vi "ChooChooLoop.vi"(8 "error in":errorcluster) -> ()   [LabVIEW 2013]
uses:
  Choo Choo State.ctl
  <vilib>/Rock Robotics/WPI/DigitalInput/WPI_DigitalInputDevRef.ctl
  <vilib>/Rock Robotics/SystemInterfaces/DIO/FPGA_DIOChannel.ctl
  <vilib>/Rock Robotics/SystemInterfaces/Typedef/FPGA_TypedefDigitalModule.ctl
  <vilib>/Rock Robotics/WPI/Encoder/WPI_EncoderDevRef.ctl
  <vilib>/Rock Robotics/SystemInterfaces/Encoder/FPGA_EncoderIdx.ctl
  <vilib>/Rock Robotics/SystemInterfaces/Counter/FPGA_CounterCtrSystemIndex.ctl
  <vilib>/Rock Robotics/WPI/Encoder/WPI_EncoderType.ctl
  <vilib>/Rock Robotics/WPI/MotorControl/WPI_MotorControlDeviceRef.ctl
  <vilib>/Rock Robotics/SystemInterfaces/DIO/FPGA_DIOPWMChannel.ctl
  <vilib>/Rock Robotics/WPI/PWM/WPI_PWMDeadband.ctl
  <vilib>/Rock Robotics/WPI/CAN/Jaguar/SubVIs/WPI_CANJaguar_ControlMode.ctl
  <vilib>/Rock Robotics/WPI/PWM/WPI_PWMTransform_ConPane.ctl
  <vilib>/Rock Robotics/WPI/Joystick/WPI_JoystickDeviceEnum.ctl
  <vilib>/Rock Robotics/WPI/SafetyOutput/WPI_SafetyOutputConfigMenu.ctl
  Robot Global Data.vi
  <vilib>/Rock Robotics/WPI/MotorControl/WPI_MotorControlSafetyCheck.vi
  <vilib>/Rock Robotics/Network Tables/SD Write String.vi
panel:
  in  "Timeout (ms)":i32=3000
  in  "Choo Choo Output":dbl=1.0
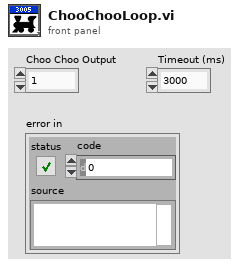
[diagram p1: front panel]
types:
  T1 = typedef "WPI_JoystickDeviceEnum.ctl" = enum16{"USB 1", "USB 2", "USB 3", "USB 4", "Kinect 1", "Kinect 2"}
  T2 = typedef "WPI_DigitalInputDevRef.ctl" = cluster{"DevStatus":errorcluster, "DIO Channel":T3, "Digital Module":T4}
  T3 = typedef "FPGA_DIOChannel.ctl" = enum8{"DIO 1", "DIO 2", "DIO 3", "DIO 4", "DIO 5", "DIO 6", "DIO 7", "DIO 8", "DIO 9", "DIO 10", "DIO 11", "DIO 12", "DIO 13", "DIO 14", "Invalid"}
  T4 = typedef "FPGA_TypedefDigitalModule.ctl" = enum16{"Digital Module 1", "Digital Module 2"}
  T5 = typedef "WPI_EncoderDevRef.ctl" = cluster{"DevStatus":errorcluster, "EncoderIndex":T6, "CounterIndex":T7, "DistancePerCount":dbl, "Decoding Type":T8}
  T6 = typedef "FPGA_EncoderIdx.ctl" = enum8{"Enc 0", "Enc 1", "Enc 2", "Enc 3", "Invalid"}
  T7 = typedef "FPGA_CounterCtrSystemIndex.ctl" = enum8{"Ctr 0", "Ctr 1", "Ctr 2", "Ctr 3", "Ctr 4", "Ctr 5", "Ctr 6", "Ctr 7", "Invalid"}
  T8 = typedef "WPI_EncoderType.ctl" = enum16{"1x", "2x", "4x"}
  T9 = typedef "WPI_MotorControlDeviceRef.ctl" = cluster{"DeviceStatus":errorcluster, "Type":enum16{"PWM", "CAN"}, "PWM":cluster{"Digital Module":T4, "PWM Channel":T10, "DeadBand":T11}, "CAN":cluster{"Device Number":u8, "Control Mode":T12, "Semaphore":T13, "Max Vout":dbl}, "Invert":bool, "TransformRef":T14, "InvTransformRef":T14}
  T10 = typedef "FPGA_DIOPWMChannel.ctl" = enum8{"PWM 1", "PWM 2", "PWM 3", "PWM 4", "PWM 5", "PWM 6", "PWM 7", "PWM 8", "PWM 9", "PWM 10", "Invalid"}
  T11 = typedef "WPI_PWMDeadband.ctl" = cluster{"Name":string, "maxPositivePwm":i32, "minPositivePwm":i32, "centerPwm":i32, "maxNegativePwm":i32, "minNegativePwm":i32, "angularRange":u16}
  T12 = typedef "WPI_CANJaguar_ControlMode.ctl" = enum8{"Percent VBus", "Current", "Speed", "Position", "Voltage"}
  T13 = typedef "Semaphore RefNum" = refnum<k1>
  T14 = typedef "WPI_PWMTransform_ConPane.ctl" = refnum<vi>
  T15 = cluster{"Ball Detect":T2, "CC Switch":T2, "Encoder":T5, "CCMotor":T9}
  T16 = typedef "Choo Choo State.ctl" = enum16{"Idle", "Check For Ball", "Drive Motor", "Delay", "Check Status", "Stop Motor"}
  T17 = typedef "WPI_JoystickDevRef.ctl" = cluster{"Device":T1}
  T18 = typedef "WPI_SafetyOutputConfigMenu.ctl" = enum16{"Enable", "Disable"}
  T19 = typedef "WPI_JoystickButtonState.ctl" = cluster{"Button 1":bool, "Button 2":bool, "Button 3":bool, "Button 4":bool, "Button 5":bool, "Button 6":bool, "Button 7":bool, "Button 8":bool, "Button 9":bool, "Button 10":bool, "Button 11":bool, "Button 12":bool}
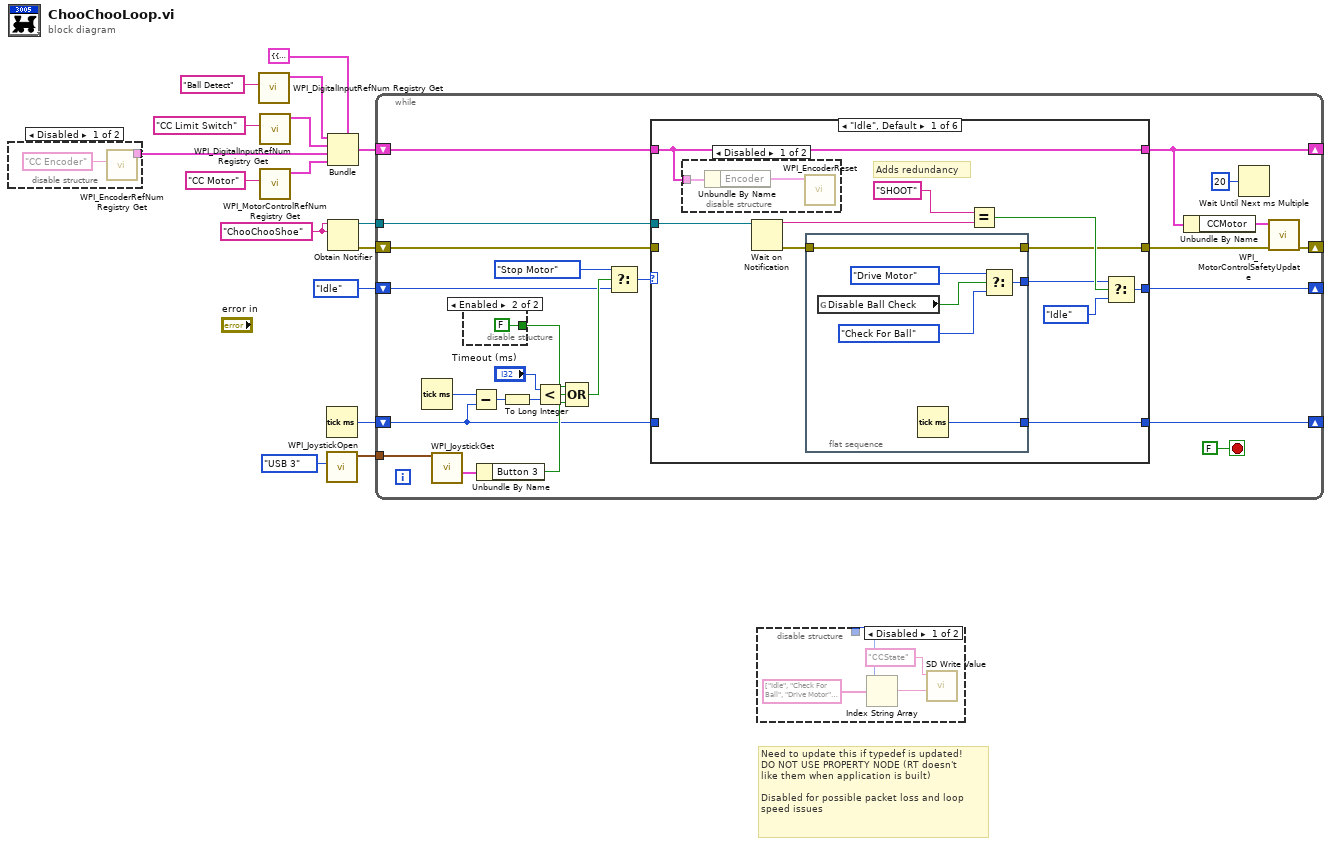
[diagram p0: block diagram]
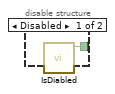
[diagram p4: hidden frame]
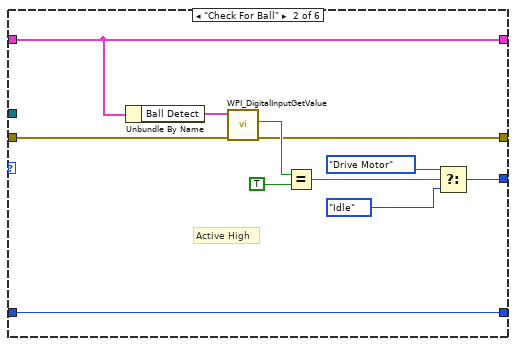
[diagram p6: hidden frame]
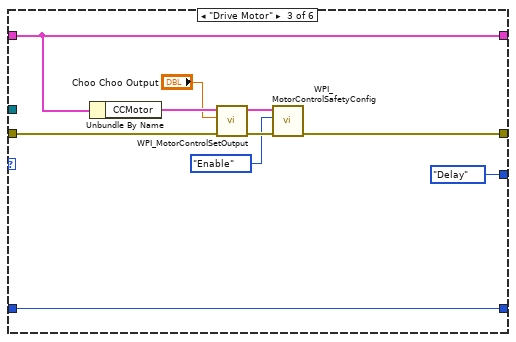
[diagram p7: hidden frame]
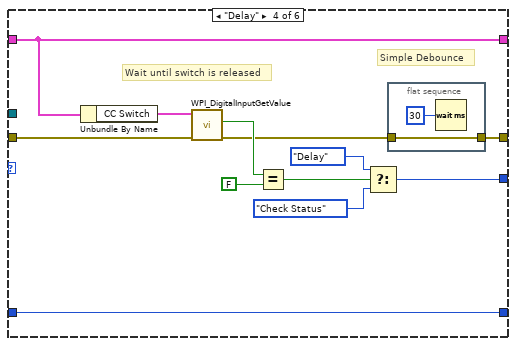
[diagram p8: hidden frame]
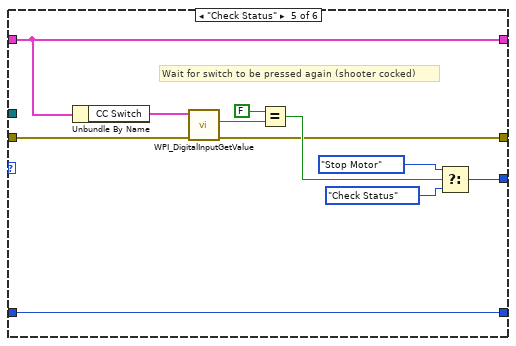
[diagram p9: hidden frame]
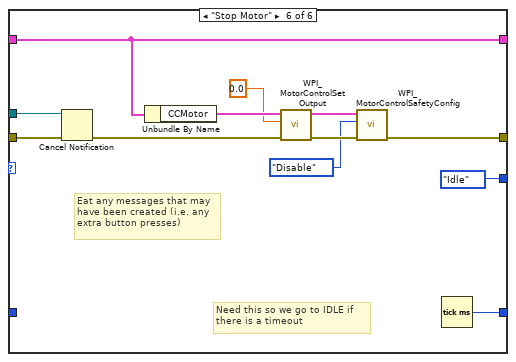
[diagram p10: hidden frame]
diagram:
  w10 = "ChooChooShoe" ("name (unnamed)")
  # "Need to update this if typedef is updated! \nDO NOT USE PROPERTY NODE (RT doesn't\nlike them when application is built)\n\nDisabled for possible packet loss and loop\nspeed issues"
  n1 = disable-structure shown="Disabled" {
    disable-tunnel: [w18 _] -> w11
    frame Disabled {
      n2 = call <vilib>:"WPI_EncoderRefNum Registry Get.vi"("refnum name"="CC Encoder") -> ("EncoderDevRef"=w18:T5)  [unwired: 9 in, 1 out]
    }
    frame Enabled {
    }
  }
  n3 = call <vilib>:"WPI_DigitalInputRefNum Registry Get.vi"("refnum name"="Ball Detect") -> ("DigitalInputDevRef"=w16:T2)  [unwired: 9 in, 1 out]
  n4 = call <vilib>:"WPI_DigitalInputRefNum Registry Get.vi"("refnum name"="CC Limit Switch") -> ("DigitalInputDevRef"=w13:T2)  [unwired: 9 in, 1 out]
  n5 = call <vilib>:"WPI_MotorControlRefNum Registry Get.vi"("refnum name"="CC Motor") -> ("MotorControlDevRef"=w9:T9)  [unwired: 9 in, 1 out]
  n6 = Tick Count (ms)() -> (millisecond timer value=w3:u32)
  n7 = call <vilib>:"WPI_JoystickOpen.vi"("JoystickDevice"=WPI_JoystickDeviceEnum."USB 3") -> ("JoystickDevRef"=w2:T17)  [unwired: 10 in]
  n8 = Bundle(cluster=T15 {"Ball Detect"={"DevStatus"={"status"=FALSE, "code"=0, "source"=""}, "DIO Channel"=enum."DIO 1", "Digital Module"=enum."Digital Module 1"}, "CC Switch"={"DevStatus"={"status"=FALSE, "code"=0, "source"=""}, "DIO Channel"=enum."DIO 1", "Digital Module"=enum."Digital Module 1"}, "Encoder"={"DevStatus"={"status"=FALSE, "code"=0, "source"=""}, "EncoderIndex"=enum."Enc 0", "CounterIndex"=enum."Ctr 0", "DistancePerCount"=0.0, "Decoding Type"=enum."1x"}, "CCMotor"={"DeviceStatus"={"status"=FALSE, "code"=0, "source"=""}, "Type"=enum."PWM", "PWM"={"Digital Module"=enum."Digital Module 1", "PWM Channel"=enum."PWM 1", "DeadBand"={"Name"="", "maxPositivePwm"=0, "minPositivePwm"=0, "centerPwm"=0, "maxNegativePwm"=0, "minNegativePwm"=0, "angularRange"=0}}, "CAN"={"Device Number"=0, "Control Mode"=enum."Percent VBus", "Semaphore"=refnum, "Max Vout"=0.0}, "Invert"=FALSE, "TransformRef"=refnum, "InvTransformRef"=refnum}}, "Ball Detect"=w16, "CC Switch"=w13, "Encoder"=w11, "CCMotor"=w9) -> (w7:T15)
  n9 = Obtain Notifier(name (unnamed)=w10, notification data type=w10) -> (notifier out=w6:refnum<notifier>, error out=w5:errorcluster)  [unwired: 2 in, 1 out]
  n10 = while {
    shift-right: [w36] -> _
    shift-left: w7 -> [w41]
    shift-right: [w33] -> _
    shift-left: Choo_Choo_State."Idle" -> [w24]
    tunnel: w6 -> [w40]
    shift-right: [w37] -> _
    shift-left: w5 -> [w39]
    shift-right: [w34] -> _
    shift-left: w3 -> [w20]
    tunnel: w2 -> [w21]
    stop <- FALSE stop-if-true
    n11 = Tick Count (ms)() -> (millisecond timer value=w31:u32)
    n12 = call <vilib>:"WPI_JoystickGet.vi"("JoystickDevRef"=w21) -> ("Buttons"=w19:T19)  [unwired: 4 in, 2 out]
    n13 = disable-structure shown="Enabled" {
      disable-tunnel: [w44 FALSE ("Is Disabled?")] -> w27
      frame Disabled {
        n14 = call "IsDiabled.vi"() -> ("Is Disabled?"=w44:bool)  [unwired: 11 in]
      }
      frame Enabled {
      }
    }
    n15 = Subtract(x=w31, y=w20) -> (x-y=w30:u32)
    n16 = Unbundle By Name(w19) -> ("Button 3"=w22:bool)
    n17 = To Long Integer(number=w30) -> (32bit integer=w25:i32)
    n18 = Less?(x="Timeout (ms)", y=w25) -> (x < y?=w28:bool)
    n19 = Compound Arithmetic op=OR(w27, w28, w22) -> (w26:bool)
    n20 = Select(t=Choo_Choo_State."Stop Motor", s=w26, f=w24) -> (s? t:f=w23:T16)
    n21 = case shown="\"Idle\", Default" w23 {
      tunnel: w41 -> [w51 w75 w85 w97 w110 w122]
      tunnel: [w51 w75 w85 w97 w110 w122] -> w36
      tunnel: w40 -> [w56 _ _ _ _ w111]
      tunnel: [w52 w70 Choo_Choo_State."Delay" w92 w103 Choo_Choo_State."Idle"] -> w33
      tunnel: [w47 w66 w78 w87 w101 w116] -> w38
      tunnel: w39 -> [_ w73 w82 w95 w102 w120]
      tunnel: w20 -> [_ w65 w76 w86 w100 _]
      tunnel: [w46 w65 w76 w86 w100 w113] -> w34
      frame "Idle", Default {
        # "Adds redundancy"
        n22 = disable-structure shown="Disabled" {
          disable-tunnel: w51 -> [w64 _]
          frame Disabled {
            n23 = Unbundle By Name(w64) -> ("Encoder"=w63:T5)
            n24 = call <vilib>:"WPI_EncoderReset.vi"("EncoderDevRef"=w63) -> ()  [unwired: 9 in, 2 out]
          }
          frame Enabled {
          }
        }
        n25 = Wait on Notification(notifier=w56) -> (notification=w54:string, error out=w48:errorcluster)  [unwired: 3 in, 2 out]
        n26 = flat-sequence {
          tunnel: [w62] -> w49
          tunnel: w48 -> [w58]
          tunnel: [w58] -> w47
          tunnel: [w57] -> w46
          frame #0 {
            n27 = global read "Robot Global Data.vi" "Disable Ball Check"() -> (w59:bool)
            n28 = Tick Count (ms)() -> (millisecond timer value=w57:u32)
            n29 = Select(t=Choo_Choo_State."Drive Motor", s=w59, f=Choo_Choo_State."Check For Ball") -> (s? t:f=w62:T16)
          }
        }
        n30 = Equal?(x="SHOOT" ("name (unnamed)"), y=w54) -> (x = y?=w53:bool)
        n31 = Select(t=w49, s=w53, f=Choo_Choo_State."Idle") -> (s? t:f=w52:T16)
      }
      frame "Check For Ball" {
        # "Active High"
        n32 = Unbundle By Name(w75) -> ("Ball Detect"=w74:T2)
        n33 = call <vilib>:"WPI_DigitalInputGetValue.vi"("error in (no error)"=w73, "DigitalInputDevRef"=w74) -> ("error out"=w66:errorcluster, "Value"=w72:bool)  [unwired: 7 in, 1 out]
        n34 = Equal?(x=w72, y=TRUE ("x")) -> (x = y?=w69:bool)
        n35 = Select(t=Choo_Choo_State."Drive Motor", s=w69, f=Choo_Choo_State."Idle") -> (s? t:f=w70:T16)
      }
      frame "Drive Motor" {
        n36 = Unbundle By Name(w85) -> ("CCMotor"=w84:T9)
        n37 = call <vilib>:"WPI_MotorControlSetOutput.vi"("error in (no error)"=w82, "Output"="Choo Choo Output", "MotorControlDevRef"=w84) -> ("error out"=w80:errorcluster, "MotorControlDevRef"=w79:T9)  [unwired: 6 in, 1 out]
        n38 = call <vilib>:"WPI_MotorControlSafetyConfig.vi"("error in (no error)"=w80, "mode"=WPI_SafetyOutputConfigMenu."Enable", "MotorControlDevRef"=w79) -> ("error out"=w78:errorcluster)  [unwired: 7 in, 1 out]
      }
      frame "Delay" {
        # "Wait until switch is released"
        # "Simple Debounce"
        n39 = Unbundle By Name(w97) -> ("CC Switch"=w96:T2)
        n40 = call <vilib>:"WPI_DigitalInputGetValue.vi"("error in (no error)"=w95, "DigitalInputDevRef"=w96) -> ("error out"=w88:errorcluster, "Value"=w94:bool)  [unwired: 7 in, 1 out]
        n41 = Equal?(x=w94, y=FALSE ("x")) -> (x = y?=w91:bool)
        n42 = Select(t=Choo_Choo_State."Delay", s=w91, f=Choo_Choo_State."Check Status") -> (s? t:f=w92:T16)
        n43 = flat-sequence {
          tunnel: w88 -> [w99]
          tunnel: [w99] -> w87
          frame #0 {
            n44 = Wait (ms)(milliseconds to wait=u32 30) -> ()  [unwired: 1 out]
          }
        }
      }
      frame "Check Status" {
        # "Wait for switch to be pressed again (shooter cocked)"
        n45 = Unbundle By Name(w110) -> ("CC Switch"=w109:T2)
        n46 = call <vilib>:"WPI_DigitalInputGetValue.vi"("error in (no error)"=w102, "DigitalInputDevRef"=w109) -> ("error out"=w101:errorcluster, "Value"=w108:bool)  [unwired: 7 in, 1 out]
        n47 = Equal?(x=FALSE ("y"), y=w108) -> (x = y?=w104:bool)
        n48 = Select(t=Choo_Choo_State."Stop Motor", s=w104, f=Choo_Choo_State."Check Status") -> (s? t:f=w103:T16)
      }
      frame "Stop Motor" {
        # "Eat any messages that may\nhave been created (i.e. any\nextra button presses)"
        # "Need this so we go to IDLE if \nthere is a timeout"
        n49 = Cancel Notification(0:w111, 3:w120) -> (11:w112:errorcluster)  [unwired: 2 out]
        n50 = Unbundle By Name(w122) -> ("CCMotor"=w121:T9)
        n51 = call <vilib>:"WPI_MotorControlSetOutput.vi"("error in (no error)"=w112, "Output"=0.0, "MotorControlDevRef"=w121) -> ("error out"=w117:errorcluster, "MotorControlDevRef"=w115:T9)  [unwired: 6 in, 1 out]
        n52 = call <vilib>:"WPI_MotorControlSafetyConfig.vi"("error in (no error)"=w117, "mode"=WPI_SafetyOutputConfigMenu."Disable", "MotorControlDevRef"=w115) -> ("error out"=w116:errorcluster)  [unwired: 7 in, 1 out]
        n53 = Tick Count (ms)() -> (millisecond timer value=w113:u32)
      }
    }
    n54 = Unbundle By Name(w36) -> ("CCMotor"=w35:T9)
    n55 = Wait Until Next ms Multiple(millisecond multiple=u32 20 ("milliseconds to wait")) -> ()  [unwired: 1 out]
    n56 = call <vilib>:"WPI_MotorControlSafetyUpdate.vi"("error in (no error)"=w38, "MotorControlDevRef"=w35) -> ("error out"=w37:errorcluster)  [unwired: 8 in, 1 out]
  }
  n57 = disable-structure shown="Disabled" {
    disable-tunnel: _ -> [w123 _]
    frame Disabled {
      n58 = Index String Array(1:w123, 2:string[] ["Idle", "Check For Ball", "Drive Motor", "Delay", "Check Status", "Stop Motor"] ("Strings []")) -> (0:w126:string)  [unwired: 1 in]
      n59 = call-poly <vilib>:"SD Write Value.vi"("String"=w126, "Name"="CCState" ("Table Prefix")) -> ()  [unwired: 8 in, 2 out]
    }
    frame Enabled {
    }
  }
